vi "Voice Level Processing.vi"(8 "error in (no error)":errorcluster, 9 "Signal Generation in":T1, 10 "Voice Level Controls in":T3, 11 "MIDI Controls in":T4=variant(dbl 0.0)) -> (0 "error out":errorcluster, 2 "Voice Level Processing out":T2)   [LabVIEW 2014, in "mySynthesizer.lvlib" / "Voice Level Processing.lvlib"]
uses:
  Voice Level Processing.lvlib
  MIDI Controls/MIDI Controls.ctl
  Voice Level Controls/Voice Level Controls.ctl
  Voice Level Processing.ctl
  Signal Generation/Signal Generation Control.ctl
  MIDI Controls/MIDI Controls.lvlib
  Voice Level Controls/Voice Level Controls.lvlib
  Signal Generation/Signal Generation.lvlib
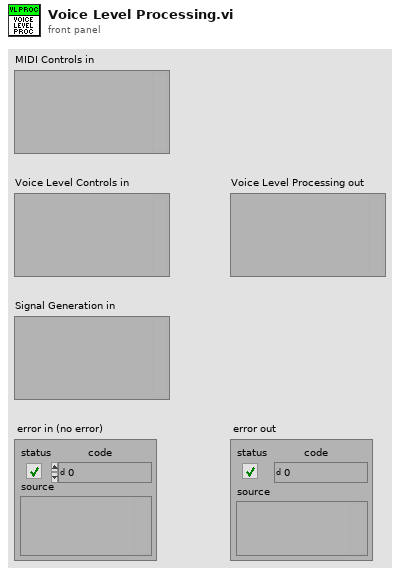
[diagram p1: front panel]
types:
  T1 = typedef "mySynthesizer.lvlib/Signal Generation.lvlib/Signal Generation Control.ctl" = variant
  T2 = typedef "mySynthesizer.lvlib/Voice Level Processing.lvlib/Voice Level Processing.ctl" = variant
  T3 = typedef "mySynthesizer.lvlib/Voice Level Controls.lvlib/Voice Level Controls.ctl" = variant
  T4 = typedef "mySynthesizer.lvlib/MIDI Controls.lvlib/MIDI Controls.ctl" = variant
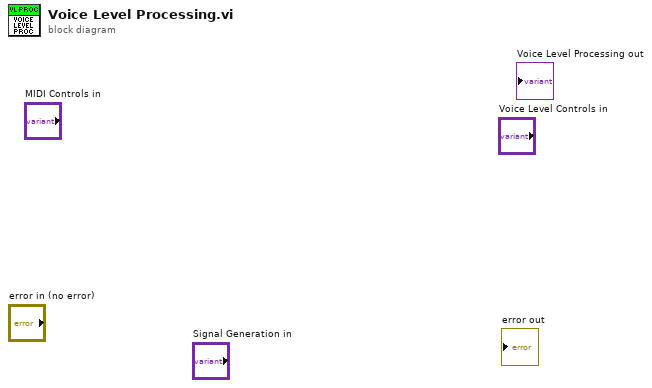
[diagram p0: block diagram]
diagram:
